vi "Passive Active, Record Results.vi"(6 "step name":string="Passive Active Waveform Parameters", 7 "Waveform Parameters":T1={"Stim Amplitude"=[], "Stim Pulse Width"=[], "Interphase Delay"=[], "Recovery Amplitude"=[], "Recovery PW"=[], "Recovery Holdoff"=[], "Frequency"=nan, "Avg CBC Width"=nan, "Avg. CBC Holdoff"=nan, "Avg. CBC Amplitude"=nan} {"Avg. CBC Amplitude" format="%.1p"; "Frequency" format="%.1p"; "Avg CBC Width" format="%.1p"; "Avg. CBC Holdoff" format="%.1p"; "Stim Pulse Width" format="%.1p"; "Interphase Delay" format="%.1p"; "Recovery PW" format="%.1p"; "Recovery Holdoff" format="%.1p"; "Stim Amplitude" format="%.1p"; "Recovery Amplitude" format="%.1p"}, 8 "error in":errorcluster, 9 "n rows":i32=21, 10 "test case":T2, 11 "Sequence Context":refnum<k7>) -> (0 "error out":errorcluster, 3 "Sequence Context dup":refnum<k7>)   [LabVIEW 2010]
doc: "This function transfers a single Compare Data Test (CDT) record to the current TestStand sequence step."
uses:
  Active Output Test Cases.ctl
  Analyze Ouptut Parameters.ctl
panel:
  in  "Acceptance Criteria":string[][](table)=[["TC16", "Pulse 1,  Stimulus Phase Amplitude", "", "4.9", "5.1", "mA", "GELE", "%.3f", "%.3f"], ["TC16", "Pulse 2,  Stimulus Phase Amplitude", "", "3.9", "4.1", "mA", "GELE", "%.3f", "%.3f"], ["TC16", "Pulse 3,  Stimulus Phase Amplitude", "", "2.9", "3.1", "mA", "GELE", "%.3f", "%.3f"], ["TC16", "Pulse 4,  Stimulus Phase Amplitude", "", "1.9", "2.1", "mA", "GELE", "%.3f", "%.3f"], ["TC16", "Pulse 1,  Stimulus Phase Pulse  Width", "", "476.000", "524.000", "us", "GELE", "%.1f", "%.1f"], ["TC16", "Pulse 2,  Stimulus Phase Pulse  Width", "", "380.000", "420.000", "us", "GELE", "%.1f", "%.1f"], ["TC16", "Pulse 3,  Stimulus Phase Pulse  Width", "", "284.000", "316.000", "us", "GELE", "%.1f", "%.1f"], ["TC16", "Pulse 4,  Stimulus Phase Pulse  Width", "", "188.000", "212.000", "us", "GELE", "%.1f", "%.1f"], ["TC16", "Pulse 1,  Active Interphase Delay", "", "93.0", "107.0", "us", "GELE", "%.1f", "%.1f"], ["TC16", "Pulse 2,  Active Interphase Delay", "", "93.0", "107.0", "us", "GELE", "%.1f", "%.1f"], ["TC16", "Pulse 3,  Active Interphase Delay", "", "93.0", "107.0", "us", "GELE", "%.1f", "%.1f"], ["TC16", "Pulse 4,  Active Interphase Delay", "", "93.0", "107.0", "us", "GELE", "%.1f", "%.1f"], ["TC16", "Pulse 1,  Passive Recovery Phase Amplitude", "", "-1.1", "-0.9", "mA", "GELE", "%.3f", "%.3f"], ["TC16", "Pulse 2,  Passive Recovery Phase Amplitude", "", "-0.9", "-0.7", "mA", "GELE", "%.3f", "%.3f"], ["TC16", "Pulse 3,  Passive Recovery Phase Amplitude", "", "-0.7", "-0.5", "mA", "GELE", "%.3f", "%.3f"], ["TC16", "Pulse 4,  Passive Recovery Phase Amplitude", "", "-0.5", "-0.3", "mA", "GELE", "%.3f", "%.3f"], ["TC16", "Pulse 1,  Passive Recovery Phase Pulse  Width", "", "2475.0", "2525.0", "us", "GELE", "%.1f", "%.1f"], ["TC16", "Pulse 2,  Passive Recovery Phase Pulse  Width", "", "1975.000", "2025.000", "us", "GELE", "%.1f", "%.1f"], ["TC16", "Pulse 3,  Passive Recovery Phase Pulse  Width", "", "1475.000", "1525.000", "us", "GELE", "%.1f", "%.1f"], ["TC16", "Pulse 4,  Passive Recovery Phase Pulse  Width", "", "975.000", "1025.000", "us", "GELE", "%.1f", "%.1f"], ["TC16", "Frequency", "", "62.725", "67.275", "Hz", "GELE", "%.3f", "%.3f"]] caption="Table 1"
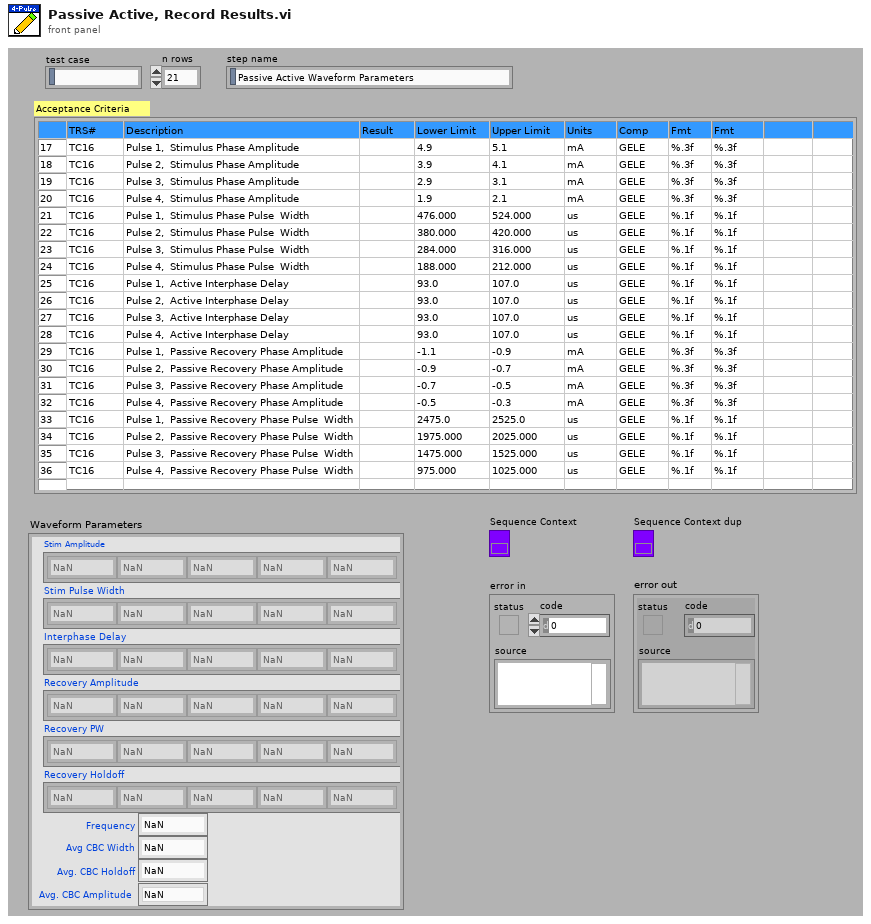
[diagram p1: front panel]
types:
  T1 = typedef "Analyze Ouptut Parameters.ctl" = cluster{"Stim Amplitude":dbl[], "Stim Pulse Width":dbl[], "Interphase Delay":dbl[], "Recovery Amplitude":dbl[], "Recovery PW":dbl[], "Recovery Holdoff":dbl[], "Frequency":dbl, "Avg CBC Width":dbl, "Avg. CBC Holdoff":dbl, "Avg. CBC Amplitude":dbl}
  T2 = typedef "Active Output Test Cases.ctl" = string
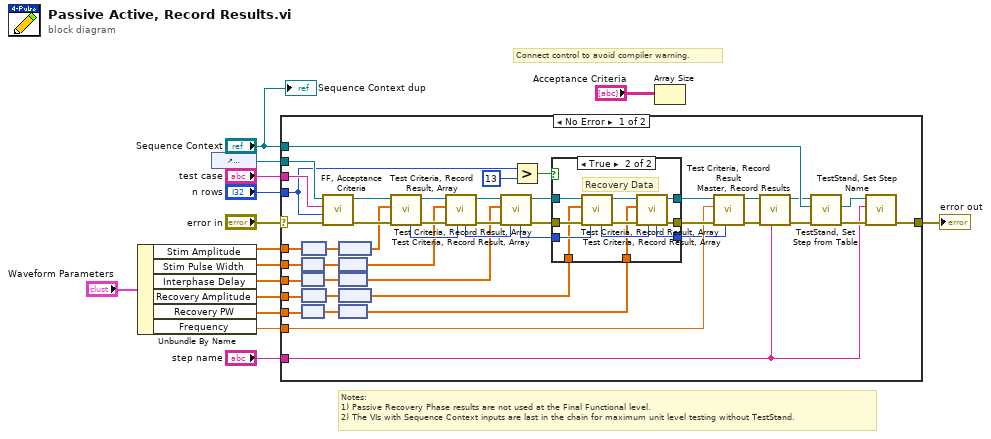
[diagram p0: block diagram]
diagram:
  # "Notes:\n1) Passive Recovery Phase results are not used at the Final Functional level.\n2) The VIs with Sequence Context inputs are last in the chain for maximum unit level testing without TestStand."
  # "Connect control to avoid compiler warning."
  n1 = Unbundle By Name("Waveform Parameters") -> ("Stim Amplitude"=w7:dbl[], "Stim Pulse Width"=w6:dbl[], "Interphase Delay"=w5:dbl[], "Recovery Amplitude"=w4:dbl[], "Recovery PW"=w3:dbl[], "Frequency"=w2:dbl)
  n2 = control-ref of="Acceptance Criteria"() -> (w10:refnum<vi>)
  n3 = case shown="No Error" "error in" {
    selector: "error in" -> [w58 w75]
    tunnel: [w56 w75] -> w15
    tunnel: "Sequence Context" -> [w55 _]
    tunnel: "test case" -> [w60 _]
    tunnel: w10 -> [w59 _]
    tunnel: "step name" -> [w16 _]
    tunnel: w2 -> [w43 _]
    tunnel: w3 -> [w37 _]
    tunnel: w4 -> [w33 _]
    tunnel: w5 -> [w34 _]
    tunnel: w6 -> [w35 _]
    tunnel: w7 -> [w42 _]
    tunnel: "n rows" -> [w23 _]
    frame No Error {
      n4 = node(w42) -> (w32:dbl[unit][])
      n5 = node(w35) -> (w31:dbl[unit][])
      n6 = node(w34) -> (w30:dbl[unit][])
      n7 = node(w33) -> (w29:dbl[unit][])
      n8 = node(w37) -> (w28:dbl[unit][])
      n9 = call "FF, Acceptance Criteria.vi"("error in"=w58, "n rows"=w23, "test case"=w60, "Tbl Refnum"=w59) -> ("error out"=w51:errorcluster, "Tbl Refnum out"=w49:refnum<vi>)  [unwired: 6 in]
      n10 = node(w32) -> (w36:dbl[])
      n11 = node(w31) -> (w27:dbl[])
      n12 = node(w30) -> (w26:dbl[])
      n13 = node(w29) -> (w25:dbl[])
      n14 = node(w28) -> (w24:dbl[])
      n15 = call "Test Criteria, Record Result, Array.vi"("error in"=w51, "Results"=w36, "Tbl Refnum"=w49) -> ("error out"=w50:errorcluster, "Tbl Refnum out"=w48:refnum<vi>, "row+n"=w41:u32)  [unwired: 6 in]
      n16 = call "Test Criteria, Record Result, Array.vi"("row (0)"=w41, "error in"=w50, "Results"=w27, "Tbl Refnum"=w48) -> ("error out"=w52:errorcluster, "Tbl Refnum out"=w47:refnum<vi>, "row+n"=w40:u32)  [unwired: 5 in]
      n17 = call "Test Criteria, Record Result, Array.vi"("row (0)"=w40, "error in"=w52, "Results"=w26, "Tbl Refnum"=w47) -> ("error out"=w53:errorcluster, "Tbl Refnum out"=w46:refnum<vi>, "row+n"=w39:u32)  [unwired: 5 in]
      n18 = Greater?(x=w23, y=13) -> (0:w21:bool)
      n19 = case shown="True" w21 {
        tunnel: w53 -> [w63 w74]
        tunnel: w46 -> [w61 w73]
        tunnel: [w63 w71] -> w45
        tunnel: [w61 w69] -> w44
        tunnel: w39 -> [w62 w68]
        tunnel: [w62 w66] -> w38
        tunnel: w25 -> [_ w65]
        tunnel: w24 -> [_ w64]
        frame False {
        }
        frame True {
          # "Recovery Data"
          n20 = call "Test Criteria, Record Result, Array.vi"("row (0)"=w68, "error in"=w74, "Results"=w65, "Tbl Refnum"=w73) -> ("error out"=w72:errorcluster, "Tbl Refnum out"=w70:refnum<vi>, "row+n"=w67:u32)  [unwired: 5 in]
          n21 = call "Test Criteria, Record Result, Array.vi"("row (0)"=w67, "error in"=w72, "Results"=w64, "Tbl Refnum"=w70) -> ("error out"=w71:errorcluster, "Tbl Refnum out"=w69:refnum<vi>, "row+n"=w66:u32)  [unwired: 5 in]
        }
      }
      n22 = call "Test Criteria, Record Result.vi"("row (0)"=w38, "error in"=w45, "Result"=w43, "Tbl Refnum"=w44) -> ("error out"=w20:errorcluster, "Tbl Refnum out"=w18:refnum<vi>)  [unwired: 5 in, 1 out]
      n23 = call "Master, Record Results.vi"("step name"=w16, "error in"=w20, "Tbl Refnum"=w18) -> ("error out"=w19:errorcluster, "Tbl Refnum dup"=w17:refnum<vi>)  [unwired: 7 in]
      n24 = call "TestStand, Set Step from Table.vi"("error in"=w19, "Sequence Context"=w55, "Tbl Refnum"=w17) -> ("error out"=w57:errorcluster, "Sequence Context Out"=w54:refnum<k7>)  [unwired: 6 in, 1 out]
      n25 = call "TestStand, Set Step Name.vi"("error in"=w57, "Step Name"=w16, "Sequence Context"=w54) -> ("error out"=w56:errorcluster)  [unwired: 7 in, 1 out]
    }
    frame Error {
    }
  }
  "error out" <- w15
  n26 = Array Size(array="Acceptance Criteria") -> ()  [unwired: 1 out]
  "Sequence Context dup" <- "Sequence Context"
